vi "test.vi"() -> ()   [LabVIEW 2020]
panel:
  out "Dark":bool
  out "Bright":bool
  out "Dim":bool
  out "Boolean 4":bool
  out "Boolean 3":bool
  in  "Boolean 2":bool
  in  "Boolean":bool
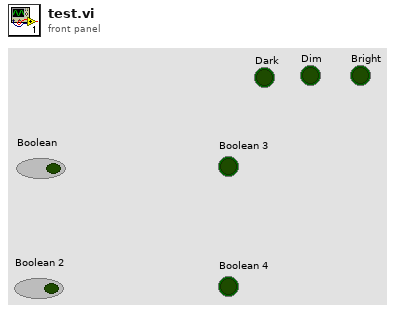
[diagram p1: front panel]
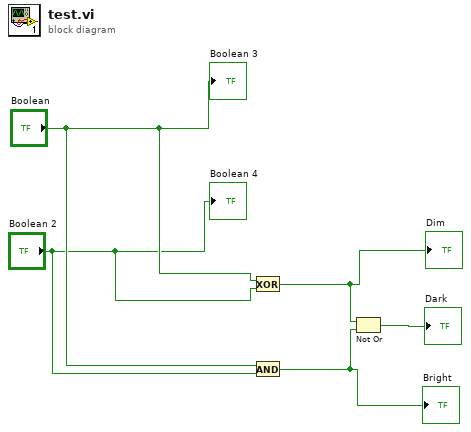
[diagram p0: block diagram]
diagram:
  n1 = Exclusive Or(1:"Boolean 2", 2:"Boolean") -> (0:w5:bool)
  "Dim" <- w5
  n2 = And(x="Boolean", y="Boolean 2") -> (x .and. y?=w4:bool)
  "Bright" <- w4
  n3 = Not Or(1:w4, 2:w5) -> (0:→"Dark":bool)
  "Boolean 3" <- "Boolean"
  "Boolean 4" <- "Boolean 2"
